vi "Calculate Forces.vi"(7 "Integrator reset":bool, 8 "error in (no error)":errorcluster, 10 "Vessel in":refnum<class "Vessel.lvclass">, 11 "PID Controller in":refnum<class "PID Controller.lvclass">) -> (0 "error out":errorcluster, 2 "Vessel out":refnum<class "Vessel.lvclass">, 3 "PID Controller out":refnum<class "PID Controller.lvclass">)   [LabVIEW 2014, in "Controller Library.lvlib" / "PID Controller.lvclass"]
doc: "This VI calculates the forces in each controlled degree of freedom direction to follow a desired path or point."
uses:
  PID Controller.lvclass
  ROV/Vessel.lvclass
  Controller.lvclass
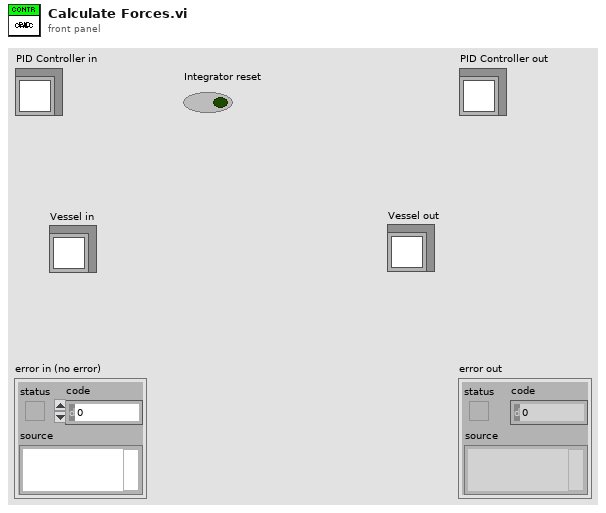
[diagram p1: front panel]
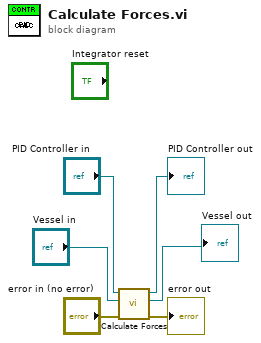
[diagram p0: block diagram]
diagram:
  n1 = call-parent "Calculate Forces.vi"("error in (no error)"="error in (no error)", "Vessel in"="Vessel in", "Controller in"="PID Controller in") -> ("error out"=→"error out":errorcluster, "Vessel out"=→"Vessel out":refnum<class "Vessel.lvclass">, "Controller out"=→"PID Controller out":refnum<class "PID Controller.lvclass">)  [unwired: 6 in]
